vi "Ship.vi"(8 "error in":errorcluster, 11 "Send MSG STEP in":refnum<class "Send MSG STEP.lvclass">) -> (0 "error out":errorcluster, 3 "Send MSG STEP out":refnum<class "Send MSG STEP.lvclass">)   [LabVIEW 2014, in "Send MSG STEP.lvlib" / "Send MSG STEP.lvclass"]
uses:
  Send MSG STEP.lvclass
  Send MSG STEP.lvclass/Send MSG STEP.ctl
  <vilib>/ActorFramework/Message Enqueuer/Message Enqueuer.lvclass/Message Enqueuer.ctl
  <vilib>/ActorFramework/Message Priority Queue/Priority Enqueue.vi
  <vilib>/ActorFramework/Message Enqueuer/Message Enqueuer.lvclass
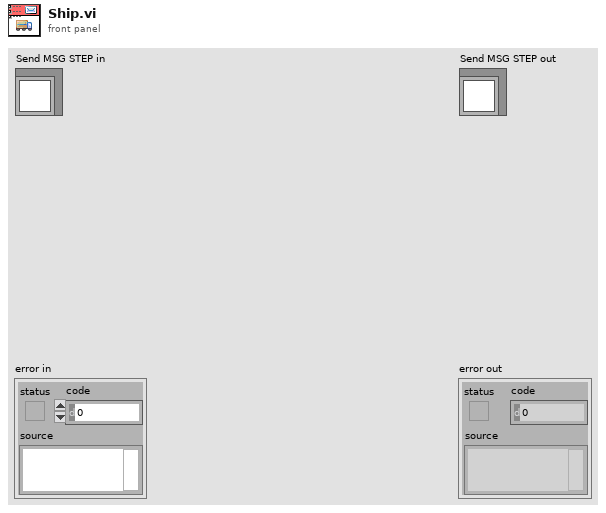
[diagram p1: front panel]
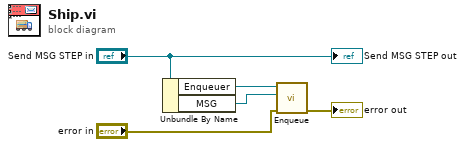
[diagram p0: block diagram]
diagram:
  n1 = Unbundle By Name("Send MSG STEP in") -> ("Enqueuer"=w4:refnum<class "Message Enqueuer.lvclass">, "MSG"=w3:refnum<class "Message.lvclass">)
  n2 = call <vilib>:"Enqueue.vi"("error in (no error)"="error in", "Message"=w3, "Message Enqueuer in"=w4) -> ("error out"=→"error out":errorcluster)  [unwired: 7 in, 1 out]
  "Send MSG STEP out" <- "Send MSG STEP in"
